vi "IPS Set Target Field.vi"(4 "Error In":errorcluster, 6 "Target Field (T)":dbl, 7 "VISA resource name":refnum<visa-resource-name>="GPIB1::25::INSTR") -> (0 "Error Out":errorcluster, 2 "Response":string, 3 "VISA resource name":refnum<visa-resource-name>)   [LabVIEW 2016, in "IPS-120.lvlib"]
uses:
  IPS-120.lvlib
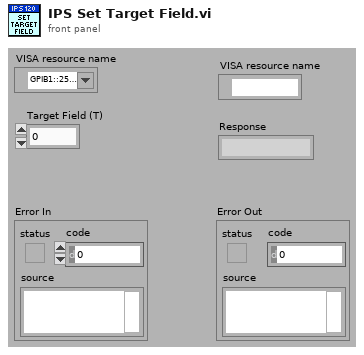
[diagram p1: front panel]
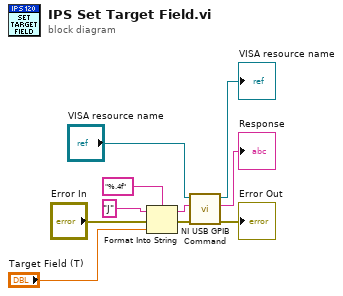
[diagram p0: block diagram]
diagram:
  n1 = Format Into String(format string="%.4f", initial string="J" ("string (\"\")"), error in="Error In", "Target Field (T)") -> (resulting string=w5:string, error out=w1:errorcluster)
  n2 = call "NI USB GPIB Command.vi"("Error In"=w1, "write buffer"=w5, "VISA resource name"="VISA resource name") -> ("Error Out"=→"Error Out":errorcluster, "read buffer"=→"Response":string, "VISA resource name out"=→"VISA resource name":refnum<visa-resource-name>)  [unwired: 6 in]
